vi "Faom Gnome Motor TestCode.vi"(10 "Step Text":string="String") -> (1 "Foam Gnome Output":string)   [LabVIEW 2014]
panel:
  in  "Foam Gnome Motor Control":dbl(slide) scale=-1.0..1.0
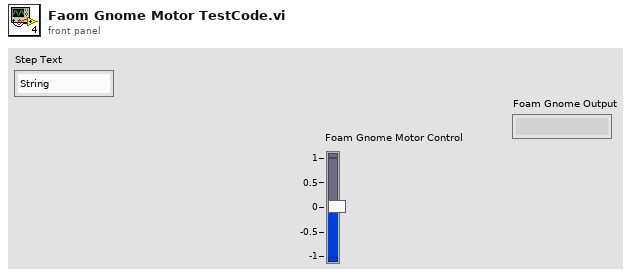
[diagram p1: front panel]
types:
  T1 = typedef "WPI_MotorControlDeviceRef.ctl" = cluster{"DeviceStatus":errorcluster, "Type":T2, "PWM":cluster{"Controller":T3, "PWM Channel":T4, "DeadBand":T5}, "CAN":cluster{"Device Number":u8, "Control Mode":T6, "Semaphore":T7, "Max Vout":dbl, "TalonSRX Control Mode":T8}, "Invert":bool, "TransformRef":T9, "InvTransformRef":T9}
  T2 = typedef "WPI_MotorControlType.ctl" = enum16{"PWM", "CAN", "CANTalonSRX"}
  T3 = typedef "FPGA_TypedefDigitalModule.ctl" = enum16{"Controller 1"}
  T4 = typedef "FPGA_DIOPWMChannel.ctl" = enum8{"PWM 0", "PWM 1", "PWM 2", "PWM 3", "PWM 4", "PWM 5", "PWM 6", "PWM 7", "PWM 8", "PWM 9", "PWM MXP 0", "PWM MXP 1", "PWM MXP 2", "PWM MXP 3", "PWM MXP 4", "PWM MXP 5", "PWM MXP 6", "PWM MXP 7", "PWM MXP 8", "PWM MXP 9", "Invalid"}
  T5 = typedef "WPI_PWMDeadband.ctl" = cluster{"Name":string, "maxPositivePwm":i32, "minPositivePwm":i32, "centerPwm":i32, "maxNegativePwm":i32, "minNegativePwm":i32, "angularRange":u16}
  T6 = typedef "WPI_CANJaguar_ControlMode.ctl" = enum8{"Percent VBus", "Current", "Speed", "Position", "Voltage"}
  T7 = typedef "Semaphore RefNum" = refnum<k1>
  T8 = typedef "WPI_CANTalonSRX_APIControlMode.ctl" = enum8{"Percent VBus", "Speed", "Position", "Slave", "Unchanged / Invalid"}
  T9 = typedef "WPI_PWMTransform_ConPane.ctl" = refnum<vi>
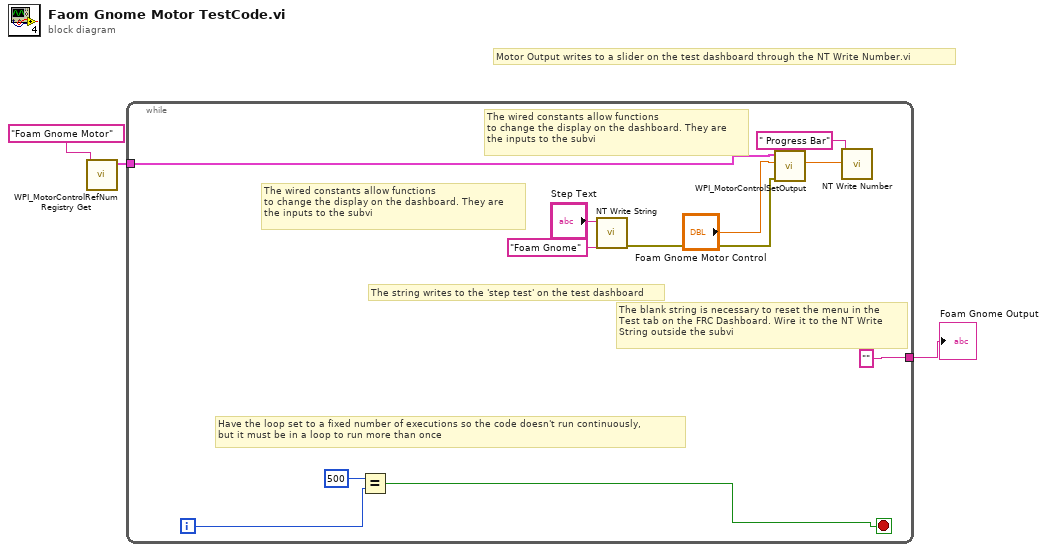
[diagram p0: block diagram]
diagram:
  # "Motor Output writes to a slider on the test dashboard through the NT Write Number.vi"
  n1 = call <vilib>:"WPI_MotorControlRefNum Registry Get.vi"("refnum name"="Foam Gnome Motor") -> ("MotorControlDevRef"=w1:T1)  [unwired: 9 in, 1 out]
  n2 = while {
    tunnel: ["" ("Drive Motors Output")] -> w3
    tunnel: w1 -> [w7]
    i -> [w6]
    stop <- w4 stop-if-true
    # "The wired constants allow functions\nto change the display on the dashboard. They are\nthe inputs to the subvi"
    # "The wired constants allow functions\nto change the display on the dashboard. They are\nthe inputs to the subvi"
    # "The string writes to the 'step test' on the test dashboard"
    # "The blank string is necessary to reset the menu in the \nTest tab on the FRC Dashboard. Wire it to the NT Write\nString outside the subvi"
    # "Have the loop set to a fixed number of executions so the code doesn't run continuously, \nbut it must be in a loop to run more than once"
    n3 = Equal?(x=500, y=w6) -> (x = y?=w4:bool)
    n4 = call <vilib>:"NT Write String.vi"("String"="Foam Gnome", "Name"="Step Text") -> ("error out"=w13:errorcluster)  [unwired: 9 in]
    n5 = call <vilib>:"WPI_MotorControlSetOutput.vi"("error in (no error)"=w13, "Output"="Foam Gnome Motor Control", "MotorControlDevRef"=w7) -> ("Motor Output"=w10:dbl)  [unwired: 6 in, 2 out]
    n6 = call <vilib>:"NT Write Number.vi"("Numeric"=w10, "Name"=" Progress Bar") -> ()  [unwired: 9 in, 1 out]
  }
  "Foam Gnome Output" <- w3
